vi "Array Manipulation.vi"() -> ()   [LabVIEW 2018]
doc: "이 VI는 다양한 배열 함수를 사용하여 데이터를 조작하는 법을 보여줍니다. 또한 LabVIEW에 포함된 다형성 기능을 사용하여 배열의 데이터를 쉽게 수정하는 방법을 보여주는 예가 들어 있습니다. \n\n다른 여러 케이스들과 블록다이어그램에 있는 주석을 통해 더 자세한 정보를 얻을 수 있습니다."
uses:
  <vilib>/measure/NI_MABase.lvlib
panel:
  in  "정지 버튼":bool
  in  "탭 컨트롤":T1(tab)
  out "연결된 데이터 배열":dbl[][](array[numeric])
  out "연결된 데이터":dbl[][](graph)
  in  "빼기?":bool
  out "데이터 배열 더하기 또는 빼기":dbl[](array[numeric])
  out "데이터 더하기 또는 빼기":dbl[](graph)
  in  "채널 선택":u16(ring) items=["채널 0", "채널 1"]
  out "단일 채널 데이터 배열":dbl[](array[numeric])
  out "단일 채널 데이터":dbl[](graph)
  out "배열의 크기":i32
  in  "오프셋":dbl(slide)=-8.326672684688674e-17 scale=-5.0..5.0
  out "웨이브폼 데이터":waveform(dbl)[](graph)
  out "데이터 채널 배열":dbl[][](array[numeric])
  in  "채널 1 오프셋":dbl(slide)=-8.326672684688674e-17 scale=-5.0..5.0
  out "모든 데이터 채널":dbl[][](graph)
  out "배열의 크기":i32[](array[numeric])
  out "데이터 배열 서브셋":dbl[][](array[numeric])
  in  "시작 값":i32(slide)=10 scale=0.0..1000.0
  out "데이터 서브셋":dbl[][](graph)
  in  "길이":i32(slide)=1000 scale=0.0..1000.0
  # "행"
  # "열"
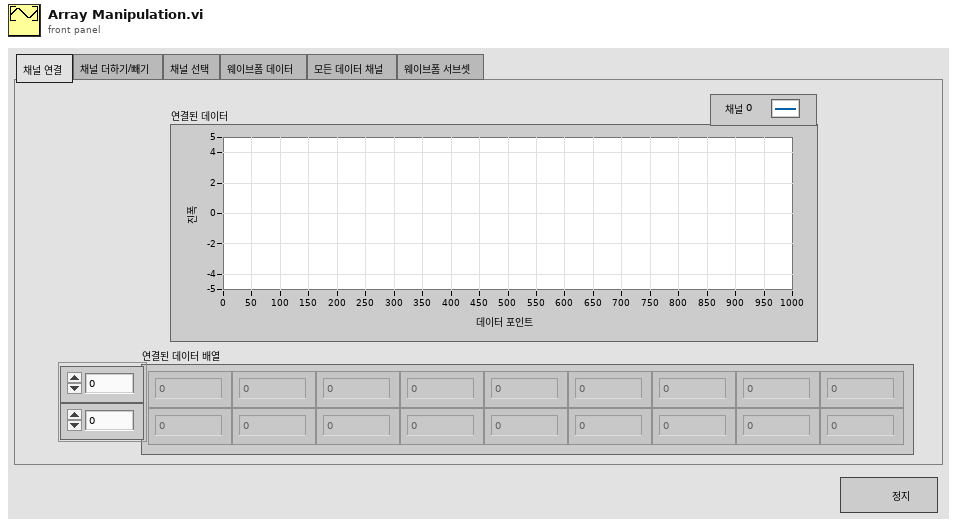
[diagram p1: front panel]
types:
  T1 = enum32{"채널 연결", "채널 더하기/빼기", "채널 선택", "웨이브폼 데이터", "모든 데이터 채널", "웨이브폼 서브셋"}
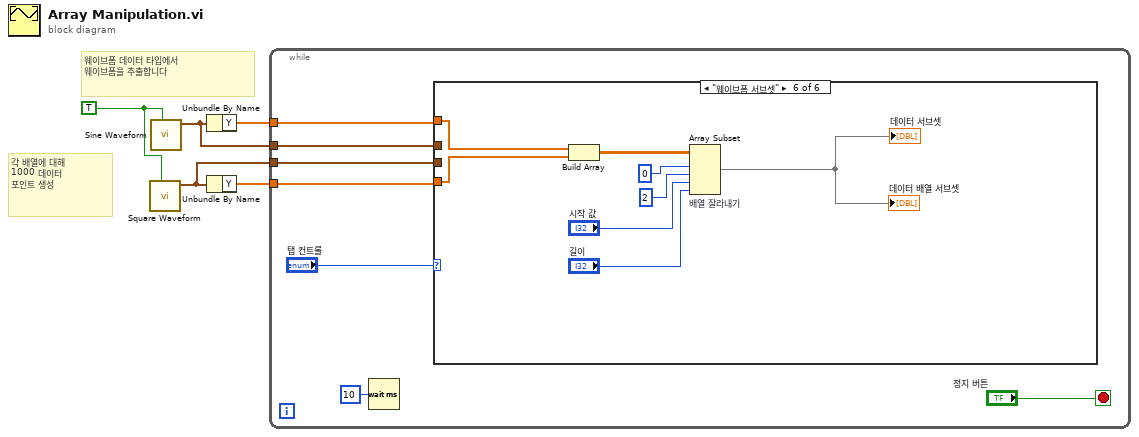
[diagram p0: block diagram]
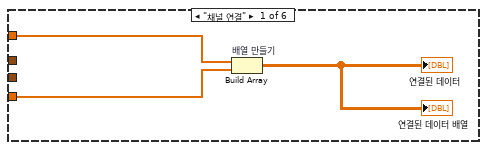
[diagram p2: hidden frame]
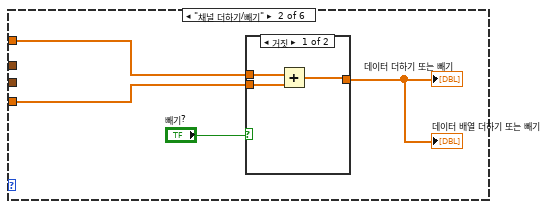
[diagram p3: hidden frame]
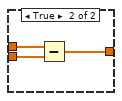
[diagram p4: hidden frame]
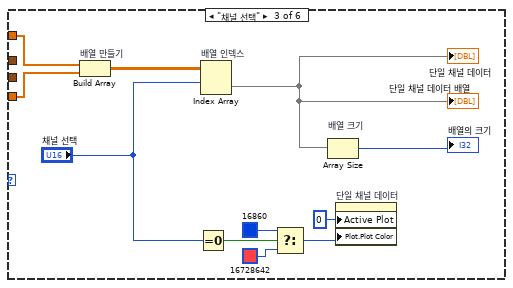
[diagram p5: hidden frame]
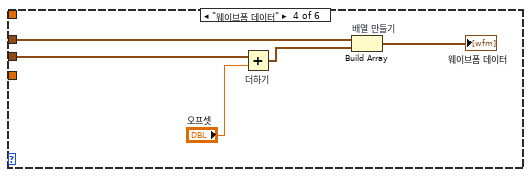
[diagram p6: hidden frame]
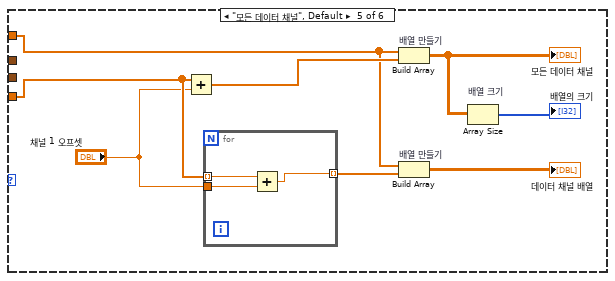
[diagram p7: hidden frame]
diagram:
  w5 = TRUE
  # "웨이브폼 데이터 타입에서\n웨이브폼을 추출합니다"
  # "각 배열에 대해\n1000 데이터\n포인트 생성"
  n1 = call <vilib>:"Square Waveform.vi"("reset signal"=w5) -> ("signal out"=w1:waveform(dbl))  [unwired: 9 in, 1 out]
  n2 = call <vilib>:"Sine Waveform.vi"("reset signal"=w5) -> ("signal out"=w2:waveform(dbl))  [unwired: 9 in, 1 out]
  n3 = Unbundle By Name ("Get Waveform Components")(w2) -> ("Y"=w4:dbl[])
  n4 = Unbundle By Name ("Get Waveform Components")(w1) -> ("Y"=w3:dbl[])
  n5 = while {
    tunnel: w4 -> [w10]
    tunnel: w3 -> [w9]
    tunnel: w2 -> [w8]
    tunnel: w1 -> [w7]
    stop <- "정지 버튼" stop-if-true
    n6 = Wait (ms)(milliseconds to wait=u32 10 ("대기 시간(ms)")) -> ()  [unwired: 1 out]
    n7 = case shown="\"웨이브폼 서브셋\"" "탭 컨트롤" {
      tunnel: w10 -> [w15 w18 w31 _ w48 w60]
      tunnel: w9 -> [w14 w17 w30 _ w43 w59]
      tunnel: w8 -> [_ _ _ w38 _ _]
      tunnel: w7 -> [_ _ _ w41 _ _]
      frame "채널 연결" {
        n8 = Build Array "배열 만들기"(w15, w14) -> (→"연결된 데이터" →"연결된 데이터 배열":dbl[][])
      }
      frame "채널 더하기/빼기" {
        n9 = case shown="거짓" "빼기?" {
          tunnel: w18 -> [w22 w25]
          tunnel: w17 -> [w21 w24]
          tunnel: [w20 w23] -> w16
          frame False {
            n10 = Add(x=w22, y=w21) -> (x+y=w20:dbl[])
          }
          frame True {
            n11 = Subtract(x=w25, y=w24) -> (x-y=w23:dbl[])
          }
        }
        "데이터 더하기 또는 빼기" <- w16
        "데이터 배열 더하기 또는 빼기" <- w16
      }
      frame "채널 선택" {
        n12 = Build Array "배열 만들기"(w31, w30) -> (w29:dbl[][])
        n13 = Equal To 0?(x="채널 선택") -> (x = 0?=w32:bool)
        n14 = Index Array "배열 인덱스"(array=w29, index (row)="채널 선택") -> (element=w27:dbl[])  [unwired: 1 in]
        "단일 채널 데이터" <- w27
        "단일 채널 데이터 배열" <- w27
        n15 = Select(t=u32 16860, s=w32, f=u32 16728642) -> (s? t:f=w35:u32)
        n16 = Array Size "배열 크기"(array=w27) -> (size(s)=→"배열의 크기":i32)
        n17 = property on="단일 채널 데이터" class="WFGraph (엄격한)"("Active Plot"=u32 0 ("활성 플롯"), "Plot.Plot Color"=w35) -> ()  [unwired: 2 in, 2 out]
      }
      frame "웨이브폼 데이터" {
        n18 = Add "더하기"(x=w41, y="오프셋") -> (x+y=w39:waveform(dbl))
        n19 = Build Array "배열 만들기"(w38, w39) -> (→"웨이브폼 데이터":waveform(dbl)[])
      }
      frame "모든 데이터 채널", Default {
        n20 = Add(x=w43, y="채널 1 오프셋") -> (x+y=w49:dbl[])
        n21 = for {
          tunnel: [w52] -> w44 mode=indexing
          tunnel: w43 -> [w51] mode=indexing
          tunnel: "채널 1 오프셋" -> [w50]
          n22 = Add(x=w51, y=w50) -> (x+y=w52:dbl)
        }
        n23 = Build Array "배열 만들기"(w48, w49) -> (w46:dbl[][])
        "모든 데이터 채널" <- w46
        n24 = Build Array "배열 만들기"(w48, w44) -> (→"데이터 채널 배열":dbl[][])
        n25 = Array Size "배열 크기"(array=w46) -> (size(s)=→"배열의 크기":i32[])
      }
      frame "웨이브폼 서브셋" {
        n26 = Build Array(w60, w59) -> (w58:dbl[][])
        n27 = Array Subset "배열 잘라내기"(array=w58, index (row)=0 ("인덱스"), length (row)=2 ("길이"), index (col)="시작 값", length (col)="길이") -> (→"데이터 배열 서브셋" →"데이터 서브셋":dbl[][])
      }
    }
  }
